vi "IO_TestLaserCnxn.vi"() -> ()   [LabVIEW 2024]
uses:
  <instrlib>/Keyence LK-G3000/Keyence LK-G3000.lvlib
panel:
  out "Numeric":i32
  out "OnLIne":bool
  out "error out":errorcluster {"code" format="%x"}
  in  "stop":bool
  out "Level PV":dbl(slide)=7.1220598220825195 scale=0.0..10.0
  out "Laser Raw":sgl=2.4953
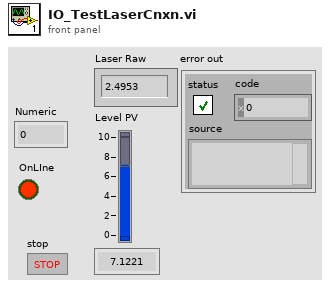
[diagram p1: front panel]
types:
  T1 = typedef "Keyence LK-G3000.lvlib/LKIF_FLOATVALUE.ctl" = cluster{"LKIF_FLOATRESULT":T2, "Value":sgl}
  T2 = typedef "Keyence LK-G3000.lvlib/LKIF_FLOATRESULT.ctl" = i32
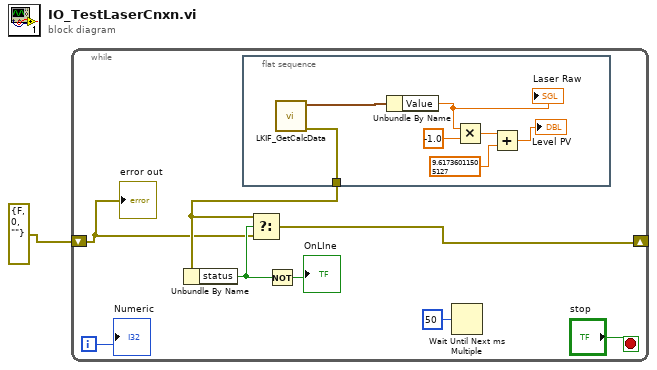
[diagram p0: block diagram]
diagram:
  n1 = while {
    shift-right: [w5] -> _
    shift-left: errorcluster {"status"=FALSE, "code"=0, "source"=""} ("error out") -> [w2]
    i -> [w6]
    stop <- "stop" stop-if-true
    n2 = Unbundle By Name(w4) -> ("status"=w3:bool)
    n3 = flat-sequence {
      tunnel: [w10] -> w4
      frame #0 {
        n4 = call <instrlib>:"LKIF_GetCalcData.vi"() -> ("error out"=w10:errorcluster, "CalcData1"=w16:T1)  [unwired: 9 in, 1 out]
        n5 = Unbundle By Name(w16) -> ("Value"=w15:sgl)
        "Laser Raw" <- w15
        n6 = Multiply(x=w15, y=sgl -1.0) -> (x*y=w13:sgl)
        n7 = Add(x=w13, y=sgl 9.61736) -> (x+y=→"Level PV":sgl)
      }
    }
    n8 = Select(t=w4, s=w3, f=w2) -> (s? t:f=w5:errorcluster)
    n9 = Not(x=w3) -> (.not. x?=→"OnLIne":bool)
    n10 = Wait Until Next ms Multiple(millisecond multiple=u32 50) -> ()  [unwired: 1 out]
    "error out" <- w2
    "Numeric" <- w6
  }
